vi "System Log JSON Consumer Loop.vi"(0 "Reactor Name":string="%y%m%d", 1 "Stop Program":refnum<vi>, 2 "date on current file":refnum<vi>, 3 "Queue JSON":refnum<vi>, 4 "Save JSON log Connection":refnum<vi>) -> ()   [LabVIEW 2021]
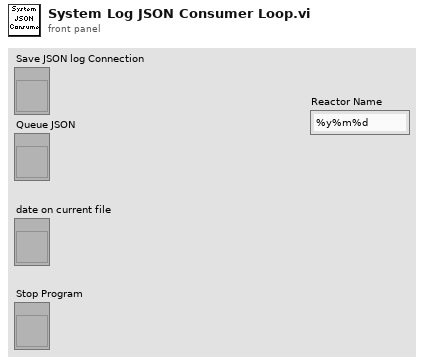
[diagram p1: front panel]
types:
  T1 = enum16{"open file", "write data", "check date", "close file"}
  T2 = enum16{"open", "replace", "create", "open or create", "replace or create", "replace or create with confirmation"}
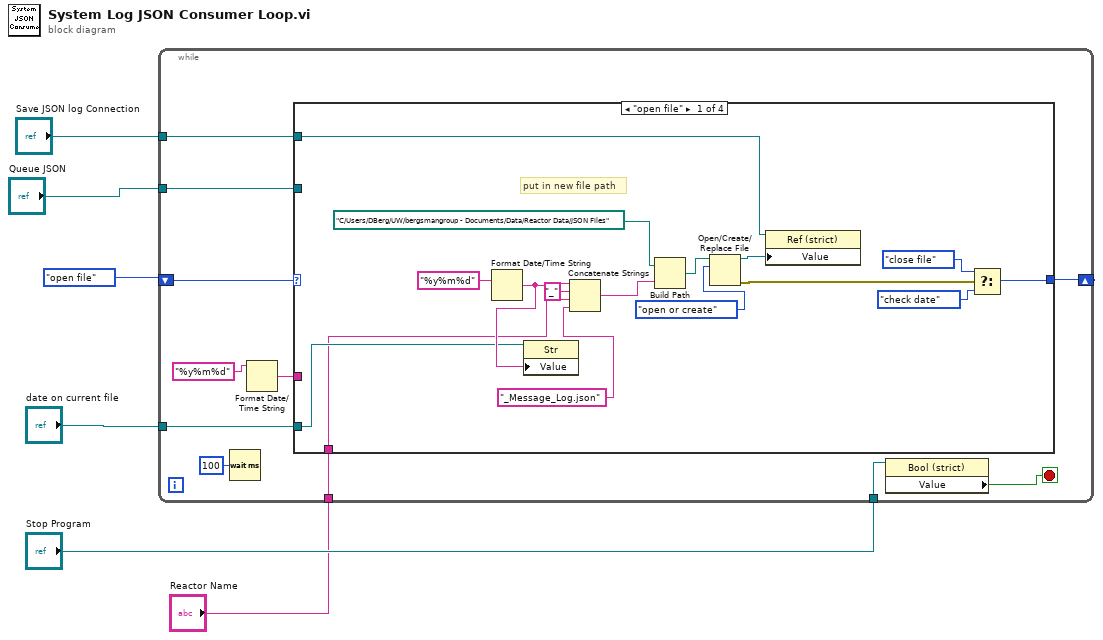
[diagram p0: block diagram]
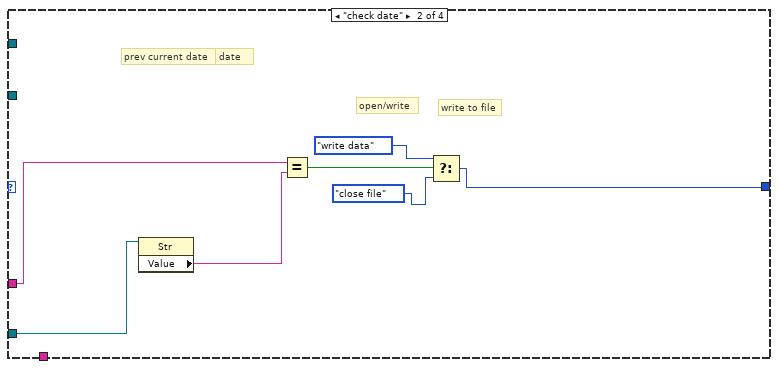
[diagram p2: hidden frame]
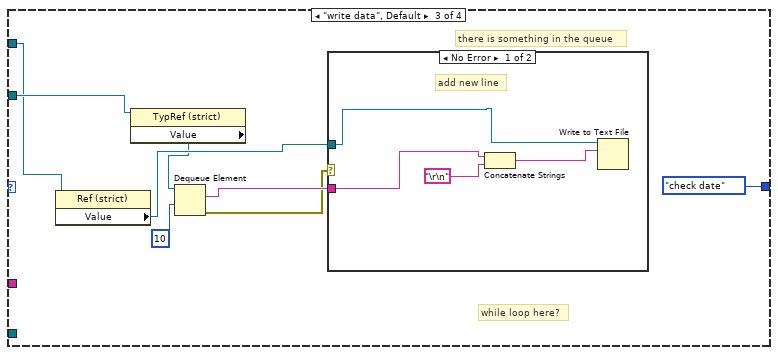
[diagram p3: hidden frame]
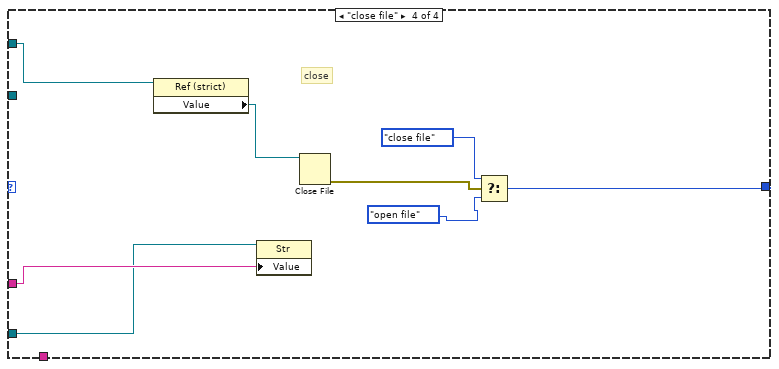
[diagram p5: hidden frame]
diagram:
  n1 = while {
    shift-right: [w16] -> _
    shift-left: T1."open file" -> [w17]
    tunnel: "date on current file" -> [w15]
    tunnel: "Save JSON log Connection" -> [w14]
    tunnel: "Queue JSON" -> [w11]
    tunnel: "Stop Program" -> [w8]
    tunnel: "Reactor Name" -> [w7]
    stop <- w9 stop-if-true
    n2 = Wait (ms)(milliseconds to wait=u32 100 ("millisecond timer value")) -> ()  [unwired: 1 out]
    n3 = Format Date/Time String(time format string (%c)="%y%m%d") -> (date/time string=w12:string)  [unwired: 2 in]
    n4 = case shown="\"open file\"" w17 {
      tunnel: [w29 w37 T1."check date" w57] -> w16
      tunnel: w15 -> [w25 w40 _ w55]
      tunnel: w14 -> [w24 _ w43 w60]
      tunnel: w12 -> [_ w36 _ w56]
      tunnel: w11 -> [_ _ w44 _]
      tunnel: w7 -> [w19 _ _ _]
      frame "open file" {
        # "put in new file path"
        n5 = Format Date/Time String(time format string (%c)="%y%m%d") -> (date/time string=w26:string)  [unwired: 2 in]
        n6 = property class="Str"(reference=w25, "Value"=w26) -> ()  [unwired: 1 in, 2 out]
        n7 = Concatenate Strings(w26, "_" ("string"), w19, "_Message_Log.json" ("time format string (%c)")) -> (w27:string)
        n8 = Build Path(base path=path "C:/Users/DBerg/UW/bergsmangroup - Documents/Data/Reactor Data/JSON Files", name or relative path=w27) -> (appended path=w33:path)
        n9 = Open/Create/Replace File(file path (use dialog)=w33, operation (0:open)=T2."open or create") -> (refnum out=w32:refnum<file>, error out=w30:errorcluster)  [unwired: 4 in, 1 out]
        n10 = property class="Ref (strict)"(reference=w24, "Value"=w32) -> ()  [unwired: 1 in, 2 out]
        n11 = Select(t=T1."close file", s=w30, f=T1."check date") -> (s? t:f=w29:T1)
      }
      frame "check date" {
        # "open/write"
        # "write to file"
        # "check most current date"
        # "prev current date"
        n12 = property class="Str"(reference=w40) -> ("Value"=w39:string)  [unwired: 1 in, 2 out]
        n13 = Equal?(x=w36, y=w39) -> (x = y?=w38:bool)
        n14 = Select(t=T1."write data", s=w38, f=T1."close file") -> (s? t:f=w37:T1)
      }
      frame "write data", Default {
        # "there is something in the queue"
        # "while loop here?"
        n15 = property class="Ref (strict)"(reference=w43) -> ("Value"=w48:refnum<file>)  [unwired: 1 in, 2 out]
        n16 = property class="TypRef (strict)"(reference=w44) -> ("Value"=w45:refnum<queue>)  [unwired: 1 in, 2 out]
        n17 = Dequeue Element(queue=w45, timeout in ms (-1)=10) -> (element=w47:string, error out=w46:errorcluster)  [unwired: 1 in, 2 out]
        n18 = case shown="No Error" w46 {
          tunnel: w47 -> [w52 _]
          tunnel: w48 -> [w50 _]
          frame No Error {
            # "add new line"
            n19 = Concatenate Strings(w52, "\r\n") -> (w51:string)
            n20 = Write to Text File(file (use dialog)=w50, text=w51) -> ()  [unwired: 2 in, 3 out]
          }
          frame Error {
          }
        }
      }
      frame "close file" {
        # "close"
        n21 = property class="Ref (strict)"(reference=w60) -> ("Value"=w59:refnum<file>)  [unwired: 1 in, 2 out]
        n22 = property class="Str"(reference=w55, "Value"=w56) -> ()  [unwired: 1 in, 2 out]
        n23 = Close File(refnum=w59) -> (error out=w58:errorcluster)  [unwired: 1 in, 1 out]
        n24 = Select(t=T1."close file", s=w58, f=T1."open file") -> (s? t:f=w57:T1)
      }
    }
    n25 = property class="Bool (strict)"(reference=w8) -> ("Value"=w9:bool)  [unwired: 1 in, 2 out]
  }
